vi "AI Timestamp Accuracy.vi"() -> ()   [LabVIEW 2020]
uses:
  9abfa4c0-cf51-4809-8978-549f57bc71e0.vi
  Utility VIs/Controls/Utilities-Wait.vi/89bc9713-8f2c-40bd-a11f-1c800a437687.vi
  <vilib>/Utility/High Resolution Relative Seconds.vi
  <vilib>/DAQmx/create/channels.llb/DAQmx Create Channel (DO-Digital Output).vi
  <vilib>/Utility/High Resolution Polling Wait.vi
  <vilib>/DAQmx/write.llb/DAQmx Write (Digital Bool 1Line 1Point).vi
  33bc07a8-6ad9-4bf6-9483-3c817cfe2bbf.vi
  <vilib>/Analysis/NI_AALPro.lvlib
  <vilib>/gmath/NI_Gmath.lvlib
  <vilib>/DAQmx/create/channels.llb/DAQmx Create Channel (AI-Voltage-Basic).vi
  <vilib>/DAQmx/configure/timing.llb/DAQmx Timing (Sample Clock).vi
  <vilib>/DAQmx/read.llb/DAQmx Read (Analog Wfm 1Chan NSamp).vi
panel:
  out "size(s)":i32
  out "Waveform Graph":dbl[](graph)
  out "median":dbl format="%.3f ms"
  out "timing":T1(graph)
  out "Iteration":i32
  out "finished":bool
  out "Graph":dbl[](graph)
  out "Array 3":dbl[](array[numeric]) format="%.6f"
  out "Array 2":dbl[](array[numeric]) format="%.6f"
  out "Array":dbl[](array[numeric]) format="%.6f"
  out "Graph":waveform(dbl)(graph)
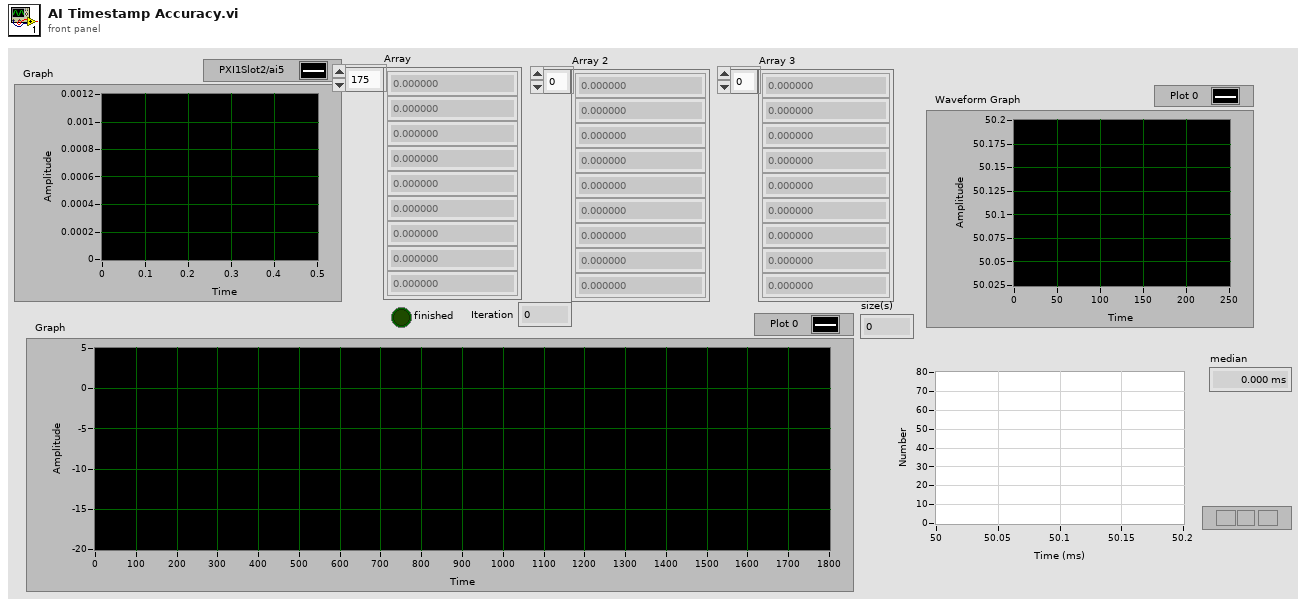
[diagram p1: front panel]
types:
  T1 = cluster{"X Values":dbl[], "Histogram: h(x)":i32[]}
  T2 = enum16{"arithmetic", "geometric", "harmonic", "trimmed", "median"}
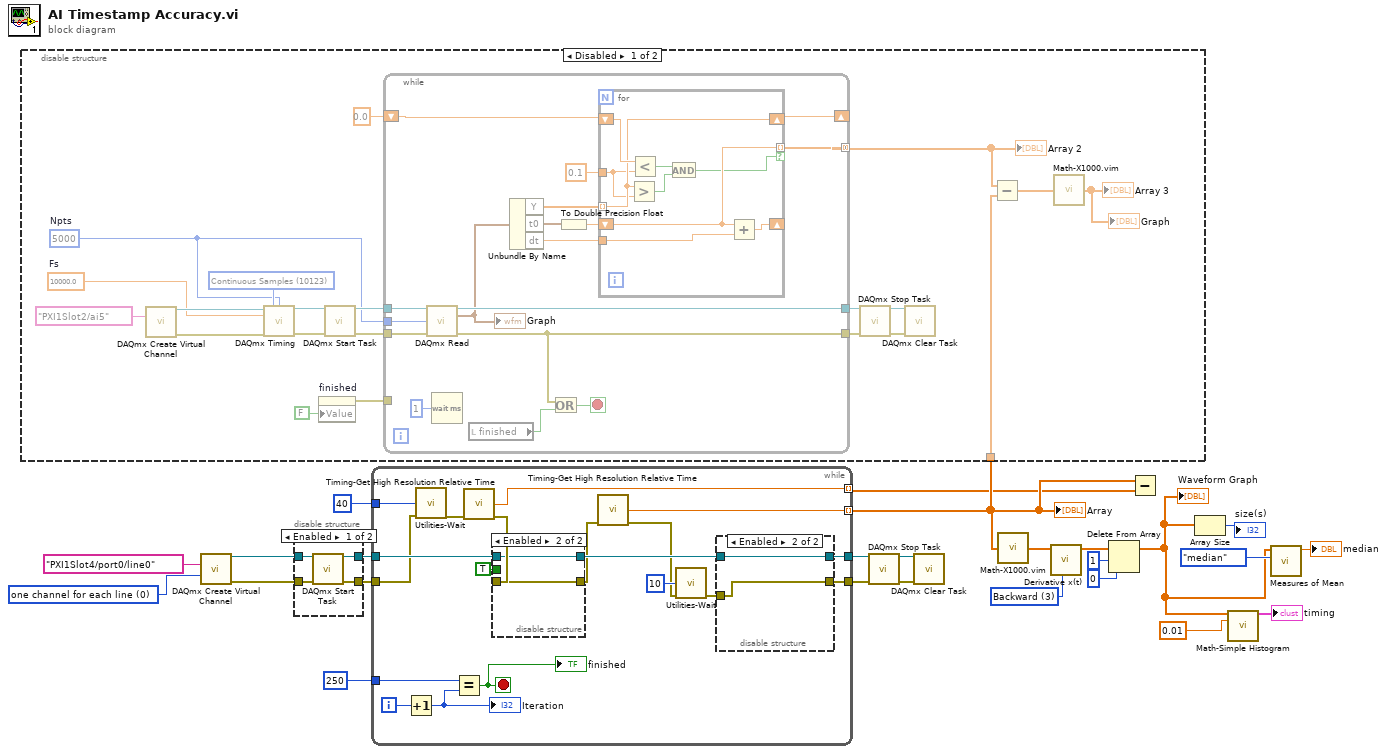
[diagram p0: block diagram]
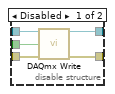
[diagram p3: hidden frame]
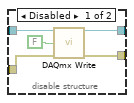
[diagram p4: hidden frame]
diagram:
  w17 = u16 3 items=["2nd Order Central", "4th Order Central", "Forward", "Backward"] ("method")
  w24 = 0 items=["one channel for each line", "one channel for all lines"] ("line grouping")
  n1 = call-poly <vilib>:"DAQmx Create Virtual Channel.vi"("lines"=tag "PXI1Slot4/port0/line0", "line grouping"=w24) -> ("task out"=w3:refnum<k21>, "error out"=w2:errorcluster)  [unwired: 12 in]
  n2 = disable-structure shown="Enabled" {
    disable-tunnel: [w29 w31] -> w5
    disable-tunnel: [w28 w30] -> w4
    disable-tunnel: w3 -> [w27 w31]
    disable-tunnel: w2 -> [w26 w30]
    frame Enabled {
      n3 = call <vilib>:"DAQmx Start Task.vi"("task/channels in"=w27, "error in"=w26) -> ("task out"=w29:refnum<k21>, "error out"=w28:errorcluster)  [unwired: 12 in]
    }
    frame Disabled {
    }
  }
  n4 = while {
    tunnel: w5 -> [w50]
    tunnel: [w46] -> w21
    tunnel: [w45] -> w20
    tunnel: [w43] -> w7 mode=indexing
    tunnel: 250 ("x") -> [w44]
    tunnel: u32 40 ("milliseconds to wait") -> [w42]
    tunnel: w4 -> [w41]
    tunnel: [w32] -> w6 mode=indexing
    i -> [w37]
    stop <- w38 stop-if-true
    n5 = Increment(x=w37) -> (x+1=w36:i32)
    "Iteration" <- w36
    n6 = call "Utilities-Wait.vi"("milliseconds to wait"=w42, "error in (no error)"=w41) -> ("error out"=w34:errorcluster)  [unwired: 13 in]
    n7 = Equal?(x=w44, y=w36) -> (x = y?=w38:bool)
    "finished" <- w38
    n8 = call "Timing-Get High Resolution Relative Time.vi"("error in (no error)"=w34) -> ("double precision float"=w32:dbl, "error out"=w33:errorcluster)  [unwired: 13 in]
    n9 = disable-structure shown="Enabled" {
      disable-tunnel: w50 -> [w55 w57]
      disable-tunnel: [w54 w57] -> w48
      disable-tunnel: [w53 w56] -> w40
      disable-tunnel: TRUE ("data") -> [w52 _]
      disable-tunnel: w33 -> [w51 w56]
      frame Disabled {
        n10 = call-poly <vilib>:"DAQmx Write.vi"("task/channels in"=w55, "data"=w52, "error in"=w51) -> ("task out"=w54:refnum<k21>, "error out"=w53:errorcluster)  [unwired: 10 in, 1 out]
      }
      frame Enabled {
      }
    }
    n11 = call "Timing-Get High Resolution Relative Time.vi"("error in (no error)"=w40) -> ("double precision float"=w43:dbl, "error out"=w39:errorcluster)  [unwired: 13 in]
    n12 = call "Utilities-Wait.vi"("milliseconds to wait"=u32 10, "error in (no error)"=w39) -> ("error out"=w47:errorcluster)  [unwired: 13 in]
    n13 = disable-structure shown="Enabled" {
      disable-tunnel: w48 -> [w62 w64]
      disable-tunnel: w47 -> [w61 w63]
      disable-tunnel: [w60 w64] -> w46
      disable-tunnel: [w59 w63] -> w45
      frame Disabled {
        n14 = call-poly <vilib>:"DAQmx Write.vi"("task/channels in"=w62, "data"=FALSE, "error in"=w61) -> ("task out"=w60:refnum<k21>, "error out"=w59:errorcluster)  [unwired: 10 in, 1 out]
      }
      frame Enabled {
      }
    }
  }
  "Array" <- w7
  n15 = disable-structure shown="Disabled" {
    disable-tunnel: w7 -> [w69 _]
    frame Disabled {
      w72 = 10000.0  # Fs
      w73 = 5000  # Npts
      w83 = 10123 items=["Finite Samples"=10178, "Continuous Samples"=10123, "Hardware Timed Single Point"=12522] ("sample mode")
      n16 = call-poly <vilib>:"DAQmx Create Virtual Channel.vi"("physical channels"=tag "PXI1Slot2/ai5") -> ("task out"=w85:refnum<k21>, "error out"=w84:errorcluster)  [unwired: 13 in]
      n17 = call-poly <vilib>:"DAQmx Timing.vi"("task/channels in"=w85, "sample mode"=w83, "samples per channel"=w73, "rate"=w72, "error in"=w84) -> ("task out"=w75:refnum<k21>, "error out"=w74:errorcluster)  [unwired: 9 in]
      n18 = property on="finished" class="Bool (strict)"("Value"=FALSE ("finished")) -> (error out=w66:errorcluster)  [unwired: 2 in, 1 out]
      n19 = call <vilib>:"DAQmx Start Task.vi"("task/channels in"=w75, "error in"=w74) -> ("task out"=w81:refnum<k21>, "error out"=w82:errorcluster)  [unwired: 12 in]
      n20 = while {
        tunnel: w82 -> [w100]
        tunnel: w81 -> [w101]
        tunnel: [w99] -> w80
        tunnel: [w97] -> w79
        tunnel: w73 -> [w98]
        shift-right: [w94] -> _
        shift-left: 0.0 -> [w95]
        tunnel: [w88] -> w70 mode=concatenating
        tunnel: w66 -> [_]
        stop <- w87 stop-if-true
        n21 = call-poly <vilib>:"DAQmx Read.vi"("task/channels in"=w101, "number of samples per channel"=w98, "error in"=w100) -> ("task out"=w99:refnum<k21>, "data"=w96:waveform(dbl), "error out"=w97:errorcluster)  [unwired: 10 in]
        "Graph" <- w96
        n22 = Wait (ms)(milliseconds to wait=u32 1) -> ()  [unwired: 1 out]
        n23 = local read "finished"() -> (w86:bool)
        n24 = Unbundle By Name(w96) -> ("Y"=w93:dbl[], "t0"=w91:timestamp, "dt"=w89:dbl)
        n25 = Or(x=w97, y=w86) -> (x .or. y?=w87:bool)
        n26 = To Double Precision Float(number=w91) -> (double precision float=w90:dbl)
        n27 = for {
          tunnel: w93 -> [w110] mode=indexing
          shift-right: [w110] -> w94
          shift-left: w95 -> [w111]
          tunnel: 0.1 -> [w109]
          tunnel: w89 -> [w105]
          shift-right: [w106] -> _
          shift-left: w90 -> [w104]
          tunnel: [w104] -> w88 mode=indexing if=w103
          n28 = Greater?(x=w110, y=w109) -> (0:w107:bool)
          n29 = Less?(x=w111, y=w109) -> (x < y?=w108:bool)
          n30 = And(x=w108, y=w107) -> (x .and. y?=w103:bool)
          n31 = Add(x=w104, y=w105) -> (x+y=w106:dbl)
        }
      }
      "Array 2" <- w70
      n32 = call <vilib>:"DAQmx Stop Task.vi"("task/channels in"=w80, "error in"=w79) -> ("task out"=w78:refnum<k21>, "error out"=w77:errorcluster)  [unwired: 12 in]
      n33 = call <vilib>:"DAQmx Clear Task.vi"("task in"=w78, "error in"=w77) -> ()  [unwired: 13 in, 1 out]
      n34 = Subtract(x=w70, y=w69) -> (x-y=w68:dbl[])
      n35 = call "Math-X1000.vim"("X"=w68) -> ("1000X"=→"Array 3" →"Graph":dbl[])
    }
    frame Enabled {
    }
  }
  n36 = call <vilib>:"DAQmx Stop Task.vi"("task/channels in"=w21, "error in"=w20) -> ("task out"=w23:refnum<k21>, "error out"=w22:errorcluster)  [unwired: 12 in]
  n37 = call <vilib>:"DAQmx Clear Task.vi"("task in"=w23, "error in"=w22) -> ()  [unwired: 13 in, 1 out]
  n38 = call "Math-X1000.vim"("X"=w7) -> ("1000X"=w13:dbl[])
  n39 = call <vilib>:"Derivative x(t).vi"("method"=w17, "X"=w13) -> ("dX/dt"=w16:dbl[])  [unwired: 8 in, 1 out]
  n40 = Delete From Array(array=w16, length=1, index=0) -> (array with subset deleted=w1:dbl[])  [unwired: 1 out]
  "Waveform Graph" <- w1
  n41 = Subtract(x=w7, y=w6) -> ()  [unwired: 1 out]
  n42 = Array Size(array=w1) -> (size(s)=→"size(s)":i32)
  n43 = call "Math-Simple Histogram.vi"("Array"=w1, "Binwidth"=0.01 ("Step")) -> ("Histogram Graph"=→"timing":T1)  [unwired: 13 in]
  n44 = call <vilib>:"Measures of Mean.vi"("type"=T2."median", "x array"=w1) -> ("mean value"=→"median":dbl)  [unwired: 8 in, 1 out]
